vi "Reset.vi"(8 "error in (no error)":errorcluster, 11 "VISA resource name":refnum<visa-resource-name>) -> (0 "error out":errorcluster, 3 "VISA resource name out":refnum<visa-resource-name>)   [LabVIEW 2020, in "GPP.lvlib"]
uses:
  GPP.lvlib
  Function/VISA_COMMON.ctl
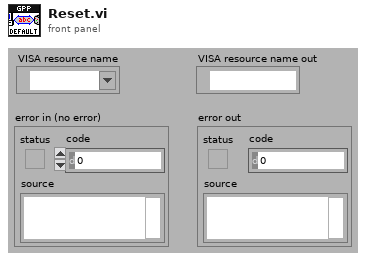
[diagram p1: front panel]
types:
  T1 = typedef "GPP.lvlib/VISA_COMMON.ctl" = enum16{"Initial", "Write CMD", "Read Result", "Read History", "Close"}
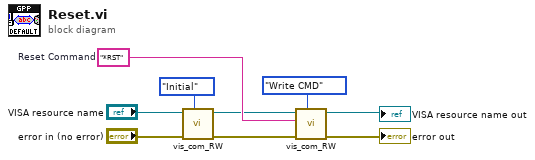
[diagram p0: block diagram]
diagram:
  w5 = "*RST"  # Reset Command
  n1 = call "vis_com_RW.vi"("Funciton"=VISA_COMMON."Initial", "error in (no error)"="error in (no error)", "VISA resource in"="VISA resource name") -> ("error out"=w4:errorcluster, "VISA resource out"=w3:refnum<visa-resource-name>)  [unwired: 6 in, 1 out]
  n2 = call "vis_com_RW.vi"("Funciton"=VISA_COMMON."Write CMD", "error in (no error)"=w4, "CMD String"=w5, "VISA resource in"=w3) -> ("error out"=→"error out":errorcluster, "VISA resource out"=→"VISA resource name out":refnum<visa-resource-name>)  [unwired: 5 in, 1 out]
